vi "Camera_Feed_ToolSelect.vi"(11 "Cropped?":bool) -> (1 "Current ROI Tool":u32, 2 "Rectangle Tool Visible?":bool, 3 "16-bit Display Mapping:Conversion Method":u32)   [LabVIEW 2024]
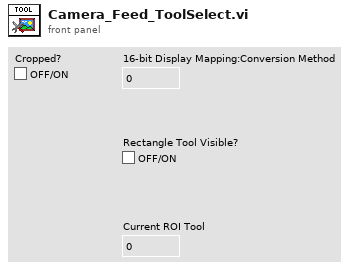
[diagram p1: front panel]
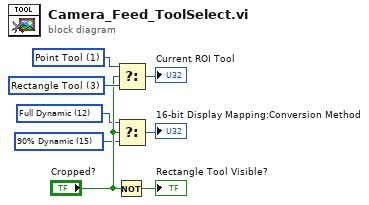
[diagram p0: block diagram]
diagram:
  w1 = u32 12 items=["Default"=10, "Most Significant Bits"=11, "Full Dynamic"=12, "Downshift"=13, "Given Range"=14, "90% Dynamic"=15, "Given Percent Range"=16] ("16-bit Display Mapping:Conversion Method")
  w2 = u32 15 items=["Default"=10, "Most Significant Bits"=11, "Full Dynamic"=12, "Downshift"=13, "Given Range"=14, "90% Dynamic"=15, "Given Percent Range"=16] ("16-bit Display Mapping:Conversion Method")
  w5 = u32 3 items=["Zoom Tool"=8, "Selection Tool"=0, "Pan Tool"=9, "Point Tool"=1, "Line Tool"=2, "Rectangle Tool"=3, "Rotated Rectangle Tool"=12, "Polyline Tool"=10, "Polygon Tool"=5, "Freehand Tool"=11, "Closed Freehand Tool"=6, "Ellipse Tool"=4, "Annulus Tool"=7] ("Current ROI Tool")
  w7 = u32 1 items=["Zoom Tool"=8, "Selection Tool"=0, "Pan Tool"=9, "Point Tool"=1, "Line Tool"=2, "Rectangle Tool"=3, "Rotated Rectangle Tool"=12, "Polyline Tool"=10, "Polygon Tool"=5, "Freehand Tool"=11, "Closed Freehand Tool"=6, "Ellipse Tool"=4, "Annulus Tool"=7] ("Current ROI Tool")
  n1 = Not(x="Cropped?") -> (.not. x?=→"Rectangle Tool Visible?":bool)
  n2 = Select(t=w7, s="Cropped?", f=w5) -> (s? t:f=→"Current ROI Tool":u32)
  n3 = Select(t=w1, s="Cropped?", f=w2) -> (s? t:f=→"16-bit Display Mapping:Conversion Method":u32)
